vi "3 Tanques.vi"() -> ()   [LabVIEW 2013]
panel:
  out "Tanque B -100":bool
  out "Tanque A -100":bool
  out "Encendido B":bool
  out "Encendido  A":bool
  out "Tank C":dbl(slide) scale=0.0..200.0
  out "Tank B":dbl(slide) scale=0.0..500.0
  out "Tank A":dbl(slide) scale=0.0..500.0
  # "Universidad De Cundinamarca\nIngenieria De sistemas \nElectiva Profesional IV\nAndy Leandro Camargo Z"
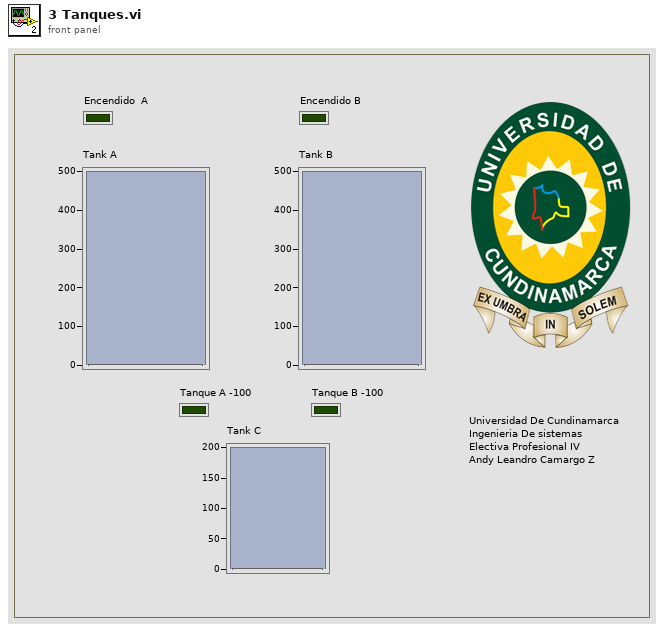
[diagram p1: front panel]
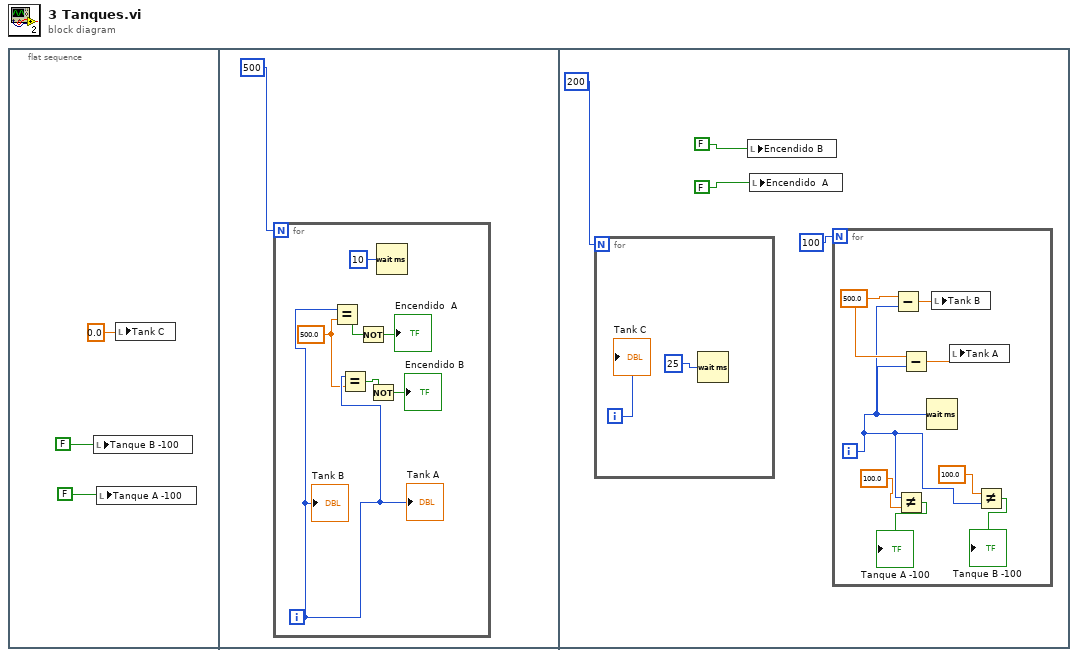
[diagram p0: block diagram]
diagram:
  n1 = flat-sequence {
    frame #0 {
      n2 = local write "Tanque B -100"(FALSE) -> ()
      n3 = local write "Tanque A -100"(FALSE) -> ()
      n4 = local write "Tank C"(0.0 ("Tank C")) -> ()
    }
    frame #1 {
      n5 = for {
        N: 500 -> [_]
        i -> [w7]
        w6 = 500.0 ("y")
        n6 = Equal?(x=w7, y=w6) -> (x = y?=w9:bool)
        n7 = Equal?(x=w7, y=w6) -> (x = y?=w5:bool)
        n8 = Not(x=w9) -> (.not. x?=→"Encendido  A":bool)
        n9 = Not(x=w5) -> (.not. x?=→"Encendido B":bool)
        n10 = Wait (ms)(milliseconds to wait=u32 10) -> ()  [unwired: 1 out]
        "Tank B" <- w7
        "Tank A" <- w7
      }
    }
    frame #2 {
      n11 = for {
        N: 200 -> [_]
        i -> [w24]
        n12 = Wait (ms)(milliseconds to wait=u32 25 ("millisecond timer value")) -> ()  [unwired: 1 out]
        "Tank C" <- w24
      }
      n13 = local write "Encendido B"(FALSE) -> ()
      n14 = local write "Encendido  A"(FALSE) -> ()
      n15 = for {
        N: 100 -> [_]
        i -> [w17]
        w21 = 500.0 ("x")
        n16 = Subtract(x=w21, y=w17) -> (x-y=w22:dbl)
        n17 = Not Equal?(x=w17, y=100.0) -> (x != y?=→"Tanque A -100":bool)
        n18 = Subtract(x=w21, y=w17) -> (x-y=w23:dbl)
        n19 = Wait (ms)(milliseconds to wait=w17) -> ()  [unwired: 1 out]
        n20 = local write "Tank B"(w22) -> ()
        n21 = local write "Tank A"(w23) -> ()
        n22 = Not Equal?(x=100.0 ("y"), y=w17) -> (x != y?=→"Tanque B -100":bool)
      }
    }
  }
